vi "RunOperation.vi"(10 "Inputs":string[](array[string]), 11 "ExecuteBuildSpec in":refnum<class "ExecuteBuildSpec.lvclass">) -> (1 "Output/Failure message":string, 2 "CLI Process Return Code":i32, 3 "ExecuteBuildSpec out":refnum<class "ExecuteBuildSpec.lvclass">)   [LabVIEW 2014, in "ExecuteBuildSpec.lvclass"]
uses:
  ExecuteBuildSpec.lvclass
  ExecuteBuildSpec.lvclass/ExecuteBuildSpec.ctl
  <vilib>/AppBuilder/AB_API_Simple/Build (path).vi
  <vilib>/AppBuilder/AB_API_Simple/NI_App_Builder_API.lvlib
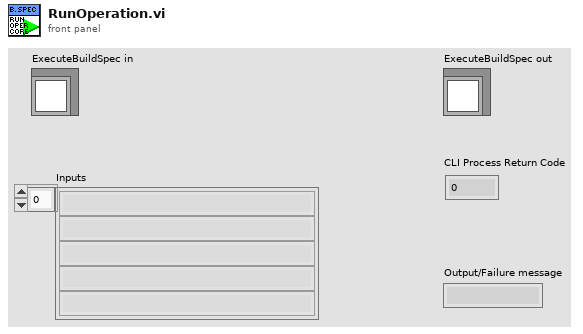
[diagram p1: front panel]
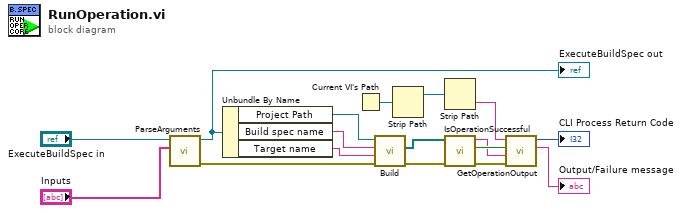
[diagram p0: block diagram]
diagram:
  n1 = call "ParseArguments.vi"("Inputs"="Inputs", "ExecuteBuildSpec in"="ExecuteBuildSpec in") -> ("error out"=w10:errorcluster, "ExecuteBuildSpec out"=w16:refnum<class "ExecuteBuildSpec.lvclass">)  [unwired: 8 in]
  "ExecuteBuildSpec out" <- w16
  n2 = Unbundle By Name(w16) -> ("Project Path"=w14:path, "Build spec name"=w13:string, "Target name"=w12:string)
  n3 = Current VI's Path() -> (path=w7:path)
  n4 = call-poly <vilib>:"Build.vi"("error in (no error)"=w10, "Name of target (My Computer)"=w12, "Name of build specification (if empty: build all)"=w13, "Path to project"=w14) -> ("error out"=w11:errorcluster, "Generated files"=w1:path[])  [unwired: 6 in]
  n5 = Strip Path(path=w7) -> (stripped path=w8:path)  [unwired: 1 out]
  n6 = Strip Path(path=w8) -> (name=w9:string)  [unwired: 1 out]
  n7 = call "IsOperationSuccessful.vi"("error in (no error)"=w11, "Generated files"=w1) -> ("error out"=w5:errorcluster, "Is Successful?"=w6:bool, "Output/Failure message"=w4:string)  [unwired: 7 in]
  n8 = call "GetOperationOutput.vi"("error in (no error)"=w5, "Operation Output/Error In"=w4, "Operation succeeded?"=w6, "Operation Name"=w9) -> ("Operation Output/Error Out"=→"Output/Failure message":string, "CLI Process Return Code"=→"CLI Process Return Code":i32)  [unwired: 6 in]
